vi "Keithley 6517A Data Format.vi"(0 "GPIB Address":string="27", 2 "Channel":bool=TRUE, 3 "Units":bool=TRUE, 4 "Status":bool=TRUE, 5 "Data Type (ASCII:0)":u16(ring) items=["ASCII", "Single Precision REAL"], 6 "External Temperature":bool, 7 "Binary Byte Order":bool, 8 "Humidity":bool, 9 "Buffered Data Elements":bool, 10 "Vsource":bool, 11 "error in (no error)":errorcluster, 13 "Reading #":bool=TRUE, 14 "TimeStamp":bool=TRUE) -> (15 "error out":T1)   [LabVIEW 2013]
doc: "This VI is used to set the data format that will be used by the 6517A to return data over the GPIB bus. Certain elements are set to ON as the default.\n\nParameters:\nGPIB Address: Default to 27\n\nData Type:\n0 = ASCII\n1 = SREAL\n\nBinary Byte Order:\nFALSE = Normal\nTRUE = Swapped\n\nChannel:\nFALSE = Off\nTRUE = On\n\nReading #:\nFALSE = Off\nTRUE = On\n\nUnits:\nFALSE = Off\nTRUE = On\n\nTimestamp:\nFALSE = Off\nTRUE = On\n\nStatus:\nFALSE = Off\nTRUE = On\n\nExternal Temperature:\nFALSE = Off\nTRUE = On\n\nHumidity:\nFALSE = Off\nTRUE = On\n\nVsource:\nFALSE = Off\nTRUE = On\n\nBuffered Data Elements:\nFALSE = No\nTRUE = YES\nSelecting YES to Buffered Data Elements\nremoves the Units and Status elements\nto be stored in the buffer."
panel:
  # "Selecting YES to Buffered Data Elements\nremoves the Units and Status elements\nto be stored in the buffer."
  # "SWAPPED\nNORMAL"
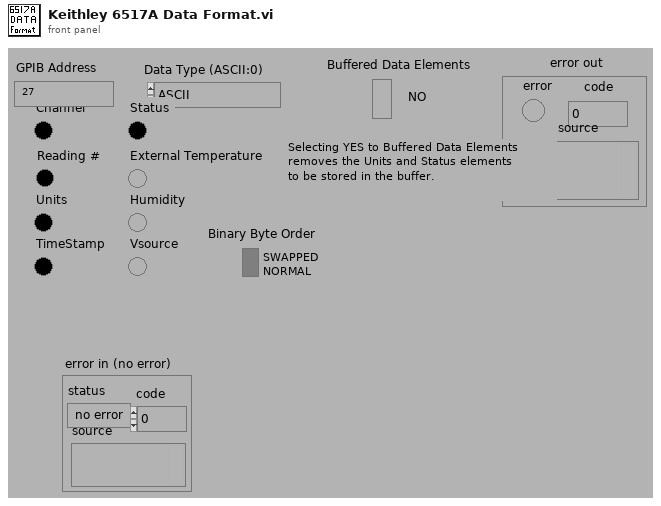
[diagram p1: front panel]
types:
  T1 = cluster{"error":bool, "code":i32, "source":string}
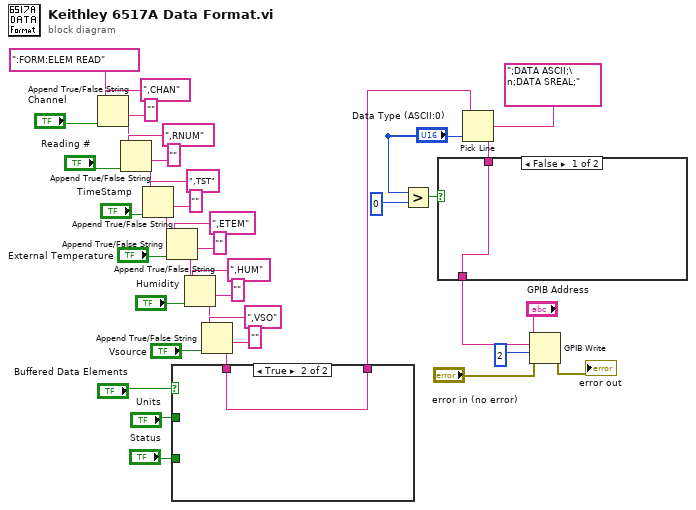
[diagram p0: block diagram]
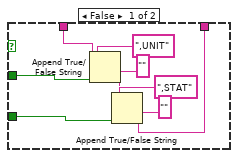
[diagram p2: hidden frame]
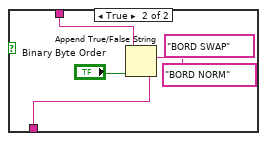
[diagram p3: hidden frame]
diagram:
  n1 = Append True/False String(1:"Channel", 2:"", 3:",CHAN", 4:":FORM:ELEM READ") -> (0:w28:string)
  n2 = Append True/False String(1:"Reading #", 2:"", 3:",RNUM", 4:w28) -> (0:w7:string)
  n3 = Append True/False String(1:"TimeStamp", 2:"", 3:",TST", 4:w7) -> (0:w6:string)
  n4 = Append True/False String(1:"External Temperature", 2:"", 3:",ETEM", 4:w6) -> (0:w14:string)
  n5 = Append True/False String(1:"Humidity", 2:"", 3:",HUM", 4:w14) -> (0:w13:string)
  n6 = Append True/False String(1:"Vsource", 2:"", 3:",VSO", 4:w13) -> (0:w4:string)
  n7 = case shown="True" "Buffered Data Elements" {
    tunnel: w4 -> [w46 w49]
    tunnel: [w42 w49] -> w3
    tunnel: "Units" -> [w41 _]
    tunnel: "Status" -> [w40 _]
    frame False {
      n8 = Append True/False String(1:w41, 2:"", 3:",UNIT", 4:w46) -> (0:w43:string)
      n9 = Append True/False String(1:w40, 2:"", 3:",STAT", 4:w43) -> (0:w42:string)
    }
    frame True {
    }
  }
  n10 = Greater?(x="Data Type (ASCII:0)", y=0) -> (0:w36:bool)
  n11 = Pick Line(string ("")=w3, multi-line string=";DATA ASCII;\n;DATA SREAL;", line index="Data Type (ASCII:0)") -> (output string=w35:string)
  n12 = case shown="False" w36 {
    tunnel: w35 -> [w50 w52]
    tunnel: [w50 w51] -> w8
    frame False {
    }
    frame True {
      n13 = Append True/False String(1:"Binary Byte Order", 2:"BORD NORM", 3:"BORD SWAP", 4:w52) -> (0:w51:string)
    }
  }
  n14 = GPIB Write(0:"GPIB Address", 1:w8, 2:2, 3:"error in (no error)") -> (6:→"error out":errorcluster)  [unwired: 1 in, 1 out]
